vi "gm_measuringpoint_valid.vi"(11 "measuring point in":u32) -> (2 "Boolean":bool, 3 "measuring point out":u32)   [LabVIEW 2011]
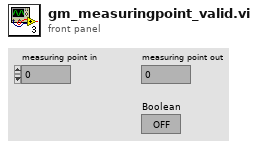
[diagram p1: front panel]
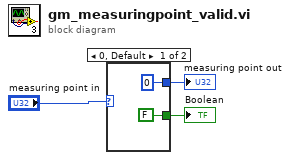
[diagram p0: block diagram]
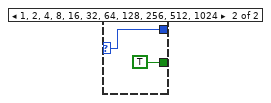
[diagram p2: hidden frame]
diagram:
  n1 = case shown="0, Default" "measuring point in" {
    selector: "measuring point in" -> [_ w7]
    tunnel: [u32 0 ("measuring point") w7] -> w2
    tunnel: [FALSE TRUE] -> w3
    frame 0, Default {
    }
    frame 1, 2, 4, 8, 16, 32, 64, 128, 256, 512, 1024 {
    }
  }
  "Boolean" <- w3
  "measuring point out" <- w2
